vi "RT Main.vi"() -> ()   [LabVIEW 2021]
panel:
  out "data received":i32[](array[numeric])
  out "#IP addresses":i32
  out "available IP addresses":string[](array[string])
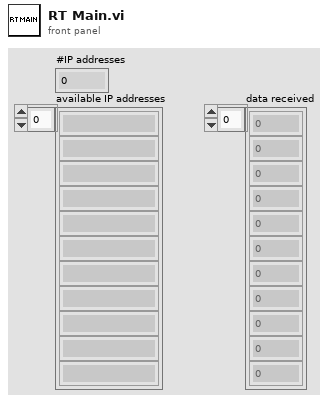
[diagram p1: front panel]
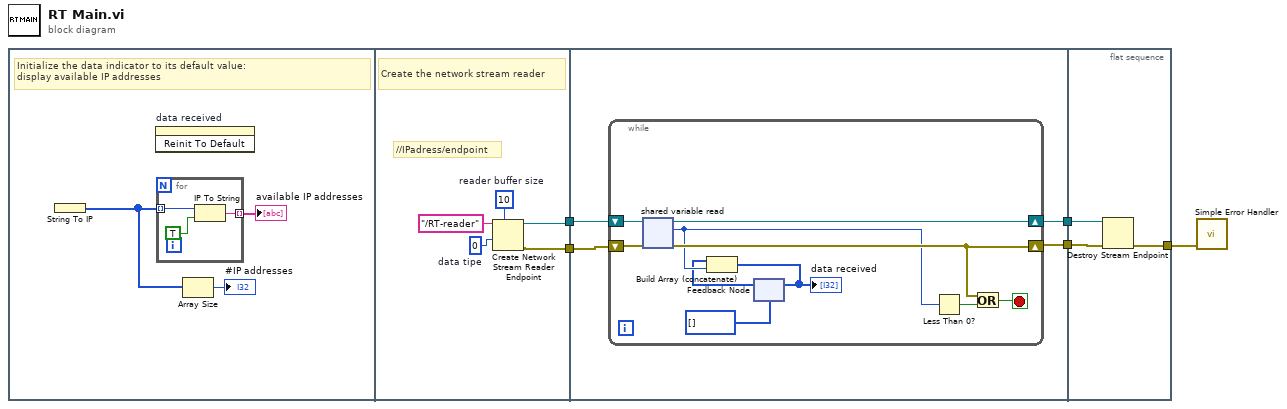
[diagram p0: block diagram]
diagram:
  n1 = flat-sequence {
    tunnel: [w13] -> w5
    tunnel: [w12] -> w4
    tunnel: w5 -> [w20]
    tunnel: w4 -> [w19]
    tunnel: [w18] -> w3
    tunnel: [w17] -> w2
    tunnel: w3 -> [w33]
    tunnel: w2 -> [w32]
    tunnel: [w31] -> w1
    frame #0 {
      # "Initialize the data indicator to its default value:\ndisplay available IP addresses"
      n2 = String To IP() -> (0:w7:u32[])  [unwired: 1 in]
      n3 = invoke on="data received" class="Arr (strict)" method="Reinit To Default"() -> ()  [unwired: 3 in, 3 out]
      n4 = for {
        tunnel: w7 -> [w10] mode=indexing
        tunnel: [w9] -> w8 mode=indexing
        n5 = IP To String(1:TRUE ("dot notation? (F)"), 2:w10) -> (0:w9:string)
      }
      "available IP addresses" <- w8
      n6 = Array Size(array=w7) -> (size(s)=→"#IP addresses":i32)
    }
    frame #1 {
      w14 = 0  # data tipe
      w16 = 10  # reader buffer size
      # "//IPadress/endpoint"
      # "Create the network stream reader"
      n7 = Create Network Stream Reader Endpoint(7:w16, 9:w14, 11:"/RT-reader" ("reader name")) -> (0:w12:errorcluster, 3:w13:refnum<k21>)  [unwired: 4 in]
    }
    frame #2 {
      n8 = while {
        shift-right: [w25] -> w17
        shift-left: w19 -> [w27]
        shift-right: [w28] -> w18
        shift-left: w20 -> [w29]
        stop <- w30 stop-if-true
        n9 = shared-variable-read(w29, w27) -> (w28:refnum<k21>, w25:errorcluster, w23:i32)  [unwired: 1 in, 1 out]
        n10 = feedback #1(i32[] [] ("data tipe")) -> (w22:i32[])
        n11 = Build Array (concatenate)(w22, w23) -> (w21:i32[])
        "data received" <- w21
        n12 = feedback-in #1(w21) -> ()
        n13 = Less Than 0?(x=w23) -> (x < 0?=w26:bool)
        n14 = Or(x=w25, y=w26) -> (x .or. y?=w30:bool)
      }
    }
    frame #3 {
      n15 = Destroy Stream Endpoint(8:w32, 11:w33) -> (0:w31:errorcluster)
    }
  }
  n16 = call <vilib>:"Simple Error Handler.vi"("error in (no error)"=w1) -> ()  [unwired: 4 in, 5 out]
